vi "Calculate Time.vi"(8 "error in (no error)":errorcluster, 11 "Controller in":refnum<class "Controller.lvclass">) -> (0 "error out":errorcluster, 3 "Controller out":refnum<class "Controller.lvclass">)   [LabVIEW 2020, in "Controller.lvclass"]
uses:
  Controller.lvclass
  Controller.lvclass/Controller.ctl
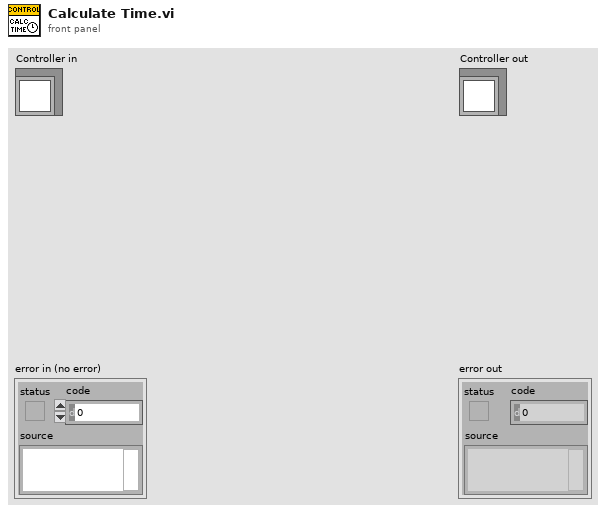
[diagram p1: front panel]
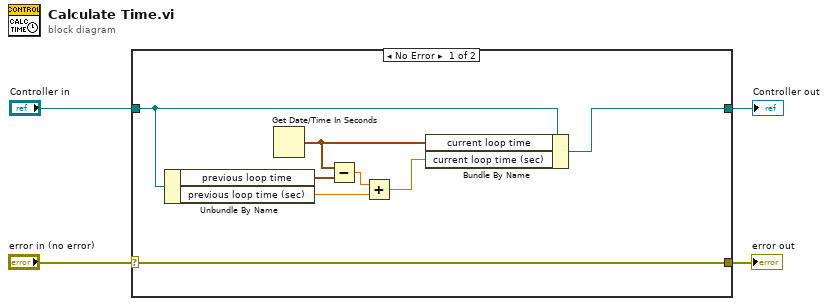
[diagram p0: block diagram]
diagram:
  n1 = case shown="No Error" "error in (no error)" {
    selector: "error in (no error)" -> [w12 w14]
    tunnel: [w12 w14] -> w3
    tunnel: [w5 w13] -> w1
    tunnel: "Controller in" -> [w8 w13]
    frame No Error {
      n2 = Unbundle By Name(w8) -> ("previous loop time"=w11:timestamp, "previous loop time (sec)"=w10:dbl)
      n3 = Get Date/Time In Seconds() -> (seconds since 1Jan1904=w7:timestamp)
      n4 = Subtract(x=w7, y=w11) -> (x-y=w9:dbl)
      n5 = Add(x=w9, y=w10) -> (x+y=w6:dbl)
      n6 = Bundle By Name(cluster=w8, "current loop time"=w7, "current loop time (sec)"=w6) -> (w5:refnum<class "Controller.lvclass">)
    }
    frame Error {
    }
  }
  "error out" <- w3
  "Controller out" <- w1
